vi "Copy Value.vi"(8 "error in (no error)":errorcluster, 10 "From":refnum<class "Type.lvclass">, 11 "Timestamp in":refnum<class "Timestamp.lvclass">) -> (0 "error out":errorcluster, 3 "Timestamp out":refnum<class "Timestamp.lvclass">)   [LabVIEW 2020, in "Conditum.lvlib" / "Columns.lvlib" / "Timestamp.lvclass"]
uses:
  Timestamp.lvclass
  Type/Type.lvclass
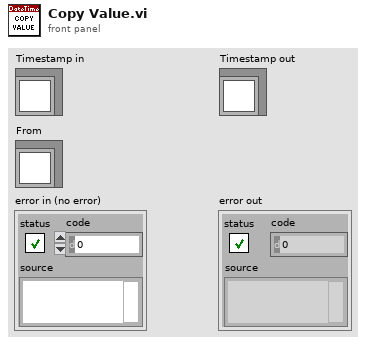
[diagram p1: front panel]
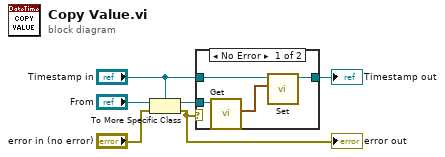
[diagram p0: block diagram]
diagram:
  n1 = To More Specific Class(target class="Timestamp in", reference="From", error in="error in (no error)") -> (specific class reference=w6:refnum<class "Timestamp.lvclass">, error out=w3:errorcluster)
  "error out" <- w3
  n2 = case shown="No Error" w3 {
    tunnel: w6 -> [w10 _]
    tunnel: "Timestamp in" -> [w8 w11]
    tunnel: [w7 w11] -> w5
    frame No Error {
      n3 = call "Get.vi"("Timestamp in"=w10) -> ("Value"=w9:timestamp)  [unwired: 10 in]
      n4 = call "Set.vi"("Time Stamp"=w9, "DateTime in"=w8) -> ("DateTime out"=w7:refnum<class "Timestamp.lvclass">)  [unwired: 9 in]
    }
    frame Error {
    }
  }
  "Timestamp out" <- w5
